vi "Configure Device.vi"(8 "error in":errorcluster, 11 "Alicat Device In":refnum<class "Alicat Device.lvclass">) -> (0 "error out":errorcluster, 3 "Alicat Device Out":refnum<class "Alicat Device.lvclass">, 4 "SP":dbl, 5 "Settable?":bool)   [LabVIEW 2015, in "Alicat Lib.lvlib" / "Alicat Device.lvclass"]
doc: "Configure the serial port for communication with the Alicat devices. We will create new Alicat objects based upon an input array of addresses. If an address is no good, then we will delete the session reference and move onto the next address. We determine if the session is good by sending a request for data to the device until the device \"wakes up\" and responds properly. If the device does not repsond properly, then set the boolean property <b>Active</b> to alert potential callers that this instantiation is non-communicative.\n\nAlthough the caller can configure the port with the desired serial and message settings, the default settings should be sufficient for most applications."
uses:
  Alicat Device.lvclass
  <vilib>/MSR Consulting, LLC/General Reuse/Session APIs/Serial/Serial Session.lvclass
  Data/Alicat Data.lvclass
  <vilib>/MSR Consulting, LLC/Configurable Device/Configurable Device.lvclass/Configurable Device.ctl
  <vilib>/MSR Consulting, LLC/General Reuse/Data/Data.lvclass/Data.ctl
  Data/Alicat Data.lvclass/Alicat Data.ctl
  Alicat Device.lvclass/Alicat Device.ctl
  <vilib>/MSR Consulting, LLC/General Reuse/Session APIs/File Access/Config Data/Config Data.lvclass/Config Data.ctl
  <vilib>/MSR Consulting, LLC/Configurable Device/Accessors/Write label.vi
  Accessors/Read Session Handle.vi
  <vilib>/MSR Consulting, LLC/Configurable Device/Read controller_.vi
  Accessors/Write Session Handle.vi
  <vilib>/MSR Consulting, LLC/Configurable Device/Accessors/Write Write Type.vi
  <vilib>/MSR Consulting, LLC/Configurable Device/Accessors/Write Config Section.vi
  <vilib>/MSR Consulting, LLC/General Reuse/Data/Write Data ID.vi
  Data/Accessors/Write ID.vi
  <vilib>/MSR Consulting, LLC/Configurable Device/Read Handle.vi
  <vilib>/MSR Consulting, LLC/Configurable Device/Read Log Session.vi
  <vilib>/Utility/config.llb/Read Key (String).vi
  <vilib>/Utility/config.llb/Read Key (Double).vi
  <vilib>/MSR Consulting, LLC/Configurable Device/Configurable Device.lvclass
  <vilib>/MSR Consulting, LLC/General Reuse/Session APIs/File Access/Config Data/Config Data.lvclass
  <vilib>/MSR Consulting, LLC/General Reuse/Session APIs/_Session Fwk/Session - Root.lvclass
  <vilib>/ErrorRing/Error Ring.xnode
  <vilib>/Utility/config.llb/NI_LVConfig.lvlib
  <vilib>/MSR Consulting, LLC/General Reuse/Session APIs/Session Log/System Log.lvclass
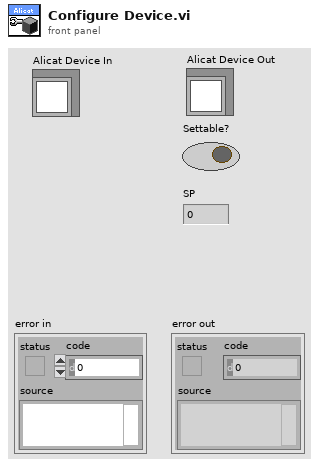
[diagram p1: front panel]
types:
  T1 = typedef "Serial Session.lvclass/Session Handle.ctl" = refnum<data-value>
  T2 = typedef "Config Data.lvclass/Config Session.ctl" = refnum<data-value>
  T3 = typedef "Session - Root.lvclass/Session Handle.ctl" = refnum<data-value>
  T4 = typedef "NI_LVConfig.lvlib/Config Data RefNum.ctl" = refnum<k1>
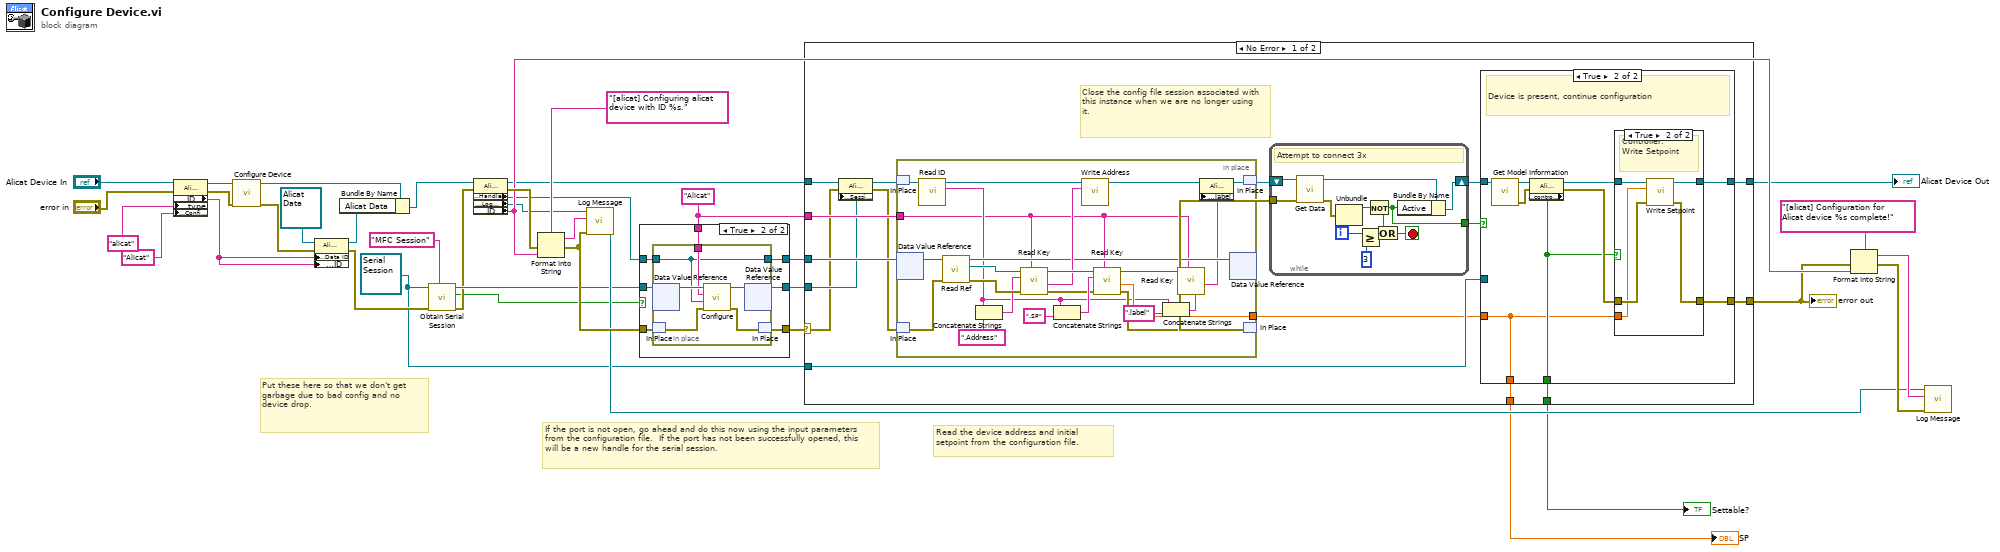
[diagram p0: block diagram]
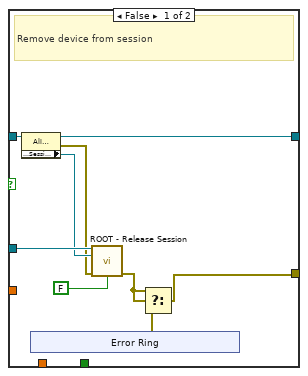
[diagram p2: hidden frame]
diagram:
  w19 = refnum<class "Serial Session.lvclass"> refnum ("Serial Session in")
  w17 = "Alicat" ("section")
  # "Put these here so that we don't get garbage due to bad config and no device drop."
  # "If the port is not open, go ahead and do this now using the input parameters from the configuration file.  If the port has not been successfully opened, this will be a new handle for the serial session."
  # "Read the device address and initial setpoint from the configuration file."
  n1 = property class="Alicat Device"(reference="Alicat Device In", error in="error in", "Accessors:type"="alicat" ("type"), "Accessors:Config Section"="Alicat" ("section")) -> (reference out=w4:refnum<class "Alicat Device.lvclass">, error out=w3:errorcluster, "Accessors:ID"=w32:string)
  n2 = call-parent "Configure Device.vi"("error in"=w3, "Device in"=w4) -> ("error out"=w2:errorcluster, "Device out"=w1:refnum<class "Alicat Device.lvclass">)  [unwired: 6 in, 2 out]
  n3 = property class="Alicat Data"(reference=refnum<class "Alicat Data.lvclass"> refnum ("Alicat Lib.lvlib:Alicat Data"), error in=w2, "Accessors:Data ID"=w32, "Accessors:ID"=w32) -> (reference out=w34:refnum<class "Alicat Data.lvclass">, error out=w35:errorcluster)
  n4 = Bundle By Name(cluster=w1, "Alicat Data"=w34) -> (w33:refnum<class "Alicat Device.lvclass">)
  n5 = call <vilib>:"Obtain Serial Session.vi"("Session Name ()"="MFC Session", "error in"=w35, "Serial Session in"=w19) -> ("error out"=w15:errorcluster, "created new?"=w12:bool, "hSerial"=w18:T1)  [unwired: 6 in]
  n6 = property class="Alicat Device"(reference=w33, error in=w15) -> (reference out=w20:refnum<class "Alicat Device.lvclass">, error out=w36:errorcluster, "Accessors:Handle"=w14:T2, "Accessors:Log Session"=w23:T3, "Accessors:ID"=w30:string)
  n7 = Format Into String(format string="[alicat] Configuring alicat device with ID %s.", error in=w36, w30) -> (resulting string=w25:string, error out=w37:errorcluster)  [unwired: 1 in]
  n8 = call <vilib>:"Log Message.vi"("error in"=w37, "MSG In"=w25, "session in"=w23) -> ("session out"=w26:T3)  [unwired: 7 in, 1 out]
  n9 = case shown="True" w12 {
    tunnel: w18 -> [w41 w48]
    tunnel: w37 -> [w40 w44]
    tunnel: [w41 w47] -> w21
    tunnel: [w40 w46] -> w22
    tunnel: w14 -> [w39 w45]
    tunnel: [w39 w43] -> w16
    tunnel: w17 -> [_ w42]
    frame False {
    }
    frame True {
      n10 = in-place {
        in-place-border: w45 -> [w49]
        in-place-border: w42 -> [w50]
        in-place-border: [w49] -> w43
        n11 = in-place-dvr #1(w48) -> (w54:refnum<class "Serial Session.lvclass">)  [unwired: 1 out]
        n12 = in-place-match #2(w44) -> (w53:errorcluster)
        n13 = call <vilib>:"Configure.vi"("error in"=w53, "Config Handle"=w49, "section"=w50, "Serial Session in"=w54) -> ("error out"=w52:errorcluster, "Serial Session out"=w51:refnum<class "Serial Session.lvclass">)  [unwired: 6 in]
        n14 = in-place-dvr #1(w51) -> (w47:T1)  [unwired: 1 out]
        n15 = in-place-match #2(w52) -> (w46:errorcluster)
      }
    }
  }
  n16 = case shown="No Error" w22 {
    selector: w22 -> [w59 w133]
    tunnel: w16 -> [w71 _]
    tunnel: w17 -> [w70 _]
    tunnel: w19 -> [w69 _]
    tunnel: [w67 w133] -> w7
    tunnel: [w64 w134] -> w8
    tunnel: w20 -> [w63 w134]
    tunnel: w21 -> [w61 _]
    tunnel: [w56 _] -> w6
    tunnel: [w55 _] -> w5
    frame No Error {
      # "Close the config file session associated with this instance when we are no longer using it."
      n17 = property class="Alicat Device"(reference=w63, error in=w59, "Accessors:Session Handle"=w61) -> (reference out=w62:refnum<class "Alicat Device.lvclass">, error out=w60:errorcluster)
      n18 = in-place {
        in-place-border: w70 -> [w109]
        in-place-border: [w121] -> w65
        n19 = in-place-match #3(w62) -> (w119:refnum<class "Alicat Device.lvclass">)
        n20 = in-place-dvr #4(w71) -> (w132:refnum<class "Config Data.lvclass">)  [unwired: 1 out]
        n21 = in-place-match #5(w60) -> (w131:errorcluster)
        n22 = call <vilib>:"Read ID.vi"("Configurable Device in"=w119) -> ("ID"=w112:string, "Configurable Device out"=w118:refnum<class "Alicat Device.lvclass">)  [unwired: 8 in, 1 out]
        n23 = call <vilib>:"Read Ref.vi"("error in"=w131, "Config Data in"=w132) -> ("error out"=w129:errorcluster, "config data"=w130:T4, "Config Data out"=w120:refnum<class "Config Data.lvclass">)  [unwired: 7 in]
        n24 = Concatenate Strings(w112, ".Address" ("string")) -> (w127:string)
        n25 = call-poly <vilib>:"Read Key.vi"("section"=w109, "error in (no error)"=w129, "key"=w127, "refnum"=w130) -> ("error out"=w123:errorcluster, "value"=w122:string, "refnum out"=w126:T4)  [unwired: 4 in, 1 out]
        n26 = Concatenate Strings(w112, ".SP" ("string")) -> (w124:string)
        n27 = call "Write Address.vi"("Address"=w122, "Alicat Device in"=w118) -> ("Alicat Device out"=w116:refnum<class "Alicat Device.lvclass">)  [unwired: 8 in, 1 out]
        n28 = call-poly <vilib>:"Read Key.vi"("section"=w109, "error in (no error)"=w123, "key"=w124, "refnum"=w126) -> ("error out"=w117:errorcluster, "value"=w121:dbl, "refnum out"=w111:T4)  [unwired: 4 in, 1 out]
        n29 = Concatenate Strings(w112, ".label" ("string")) -> (w113:string)
        n30 = call-poly <vilib>:"Read Key.vi"("section"=w109, "key"=w113, "refnum"=w111) -> ("value"=w110:string)  [unwired: 5 in, 3 out]
        n31 = property class="Alicat Device"(reference=w116, "Accessors:label"=w110) -> (reference out=w115:refnum<class "Alicat Device.lvclass">)  [unwired: 1 in, 1 out]
        n32 = in-place-dvr #4(w120) -> ()  [unwired: 2 out]
        n33 = in-place-match #3(w115) -> (w68:refnum<class "Alicat Device.lvclass">)
        n34 = in-place-match #5(w117) -> (w57:errorcluster)
      }
      n35 = while {
        tunnel: w57 -> [w103]
        shift-right: [w101] -> w66
        shift-left: w68 -> [w104]
        tunnel: [w100] -> w58
        i -> [w98]
        stop <- w105 stop-if-true
        # "Attempt to connect 3x"
        n36 = call-dynamic "Get Data.vi"("error in"=w103, "Alicat Device in"=w104) -> ("error out"=w99:errorcluster, "Alicat Device out"=w102:refnum<class "Alicat Device.lvclass">)  [unwired: 7 in, 1 out]
        n37 = Unbundle(w99) -> ("status"=w106:bool)  [unwired: 2 out]
        n38 = Greater Or Equal?(x=w98, y=3) -> (x >= y?=w107:bool)
        n39 = Not(x=w106) -> (.not. x?=w100:bool)
        n40 = Or(x=w100, y=w107) -> (x .or. y?=w105:bool)
        n41 = Bundle By Name(cluster=w102, "Active"=w100) -> (w101:refnum<class "Alicat Device.lvclass">)
      }
      n42 = case shown="True" w58 {
        tunnel: [w72 w89] -> w67
        tunnel: w69 -> [w80 _]
        tunnel: w66 -> [w78 w90]
        tunnel: w65 -> [_ w82]
        tunnel: [w77 w88] -> w64
        tunnel: [_ w83] -> w56
        tunnel: [_ w82] -> w55
        frame False {
          # "Remove device from session"
          n43 = property class="Alicat Device"(reference=w78) -> (reference out=w77:refnum<class "Alicat Device.lvclass">, error out=w75:errorcluster, "Accessors:Session Handle"=w76:T1)  [unwired: 1 in]
          n44 = xnode "Error Ring"() -> ("error out"=w73:errorcluster)
          n45 = call <vilib>:"ROOT - Release Session.vi"("OBJ - Session in"=w80, "Session Handle in"=w76, "error in (no error)"=w75, "force destroy? (F)"=FALSE) -> ("error out"=w74:errorcluster)  [unwired: 10 in, 1 out]
          n46 = Select(t=w74, s=w74, f=w73) -> (s? t:f=w72:errorcluster)
        }
        frame True {
          # "Device is present, continue configuration"
          n47 = call "Get Model Information.vi"("Alicat Device in"=w90) -> ("error out"=w84:errorcluster, "Alicat Device out"=w87:refnum<class "Alicat Device.lvclass">)  [unwired: 7 in, 2 out]
          n48 = property class="Alicat Device"(reference=w87, error in=w84) -> (reference out=w86:refnum<class "Alicat Device.lvclass">, error out=w85:errorcluster, "Accessors:controller_"=w83:bool)
          n49 = case shown="True" w83 {
            tunnel: w85 -> [w91 w96]
            tunnel: w86 -> [w92 w97]
            tunnel: w82 -> [_ w93]
            tunnel: [w91 w95] -> w89
            tunnel: [w92 w94] -> w88
            frame False {
            }
            frame True {
              # "Controller:\nWrite Setpoint"
              n50 = call "Write Setpoint.vi"("error in"=w96, "Setpoint"=w93, "Alicat Device in"=w97) -> ("error out"=w95:errorcluster, "Alicat Device out"=w94:refnum<class "Alicat Device.lvclass">)  [unwired: 6 in, 1 out]
            }
          }
        }
      }
    }
    frame Error {
    }
  }
  "error out" <- w7
  "Alicat Device Out" <- w8
  "Settable?" <- w6
  "SP" <- w5
  n51 = Format Into String(format string="[alicat] Configuration for Alicat device %s complete!", error in=w7, w30) -> (resulting string=w28:string, error out=w29:errorcluster)  [unwired: 1 in]
  n52 = call <vilib>:"Log Message.vi"("error in"=w29, "MSG In"=w28, "session in"=w26) -> ()  [unwired: 7 in, 2 out]
